vi "LinearQuadraticRegulator_Calculate_NextR.vi"(9 "NextR":T1, 10 "X":T1, 11 "in LinearQuadraticRegulator":T2) -> (0 "Error":bool, 2 "U":T1, 3 "out LinearQuadraticRegulator":T2)   [LabVIEW 2019, in "Trajectory_Library.lvlib"]
doc: "Creates a new LINEAR SYSTEM data cluster with the specified values. \n\n\nInputs: \n - XXX -- XXX.\n\nOutputs:\n - XXX -- XXX."
uses:
  Trajectory_Library.lvlib
  LINEAR_QUADRATIC_REGULATOR.ctl
  <vilib>/Analysis/Matrix/Datatypes/RealMatrix.ctl
  <vilib>/Analysis/Matrix/NI_Matrix.lvlib
panel:
  # "Ref State <States,1>"
  # "Comp and capped \noutput <Inputs,1>"
  # "Controller gain\n<Inputs,States>"
  # "Ref State <States,1>"
  # "Comp and capped \noutput <Inputs,1>"
  # "Controller gain\n<Inputs,States>"
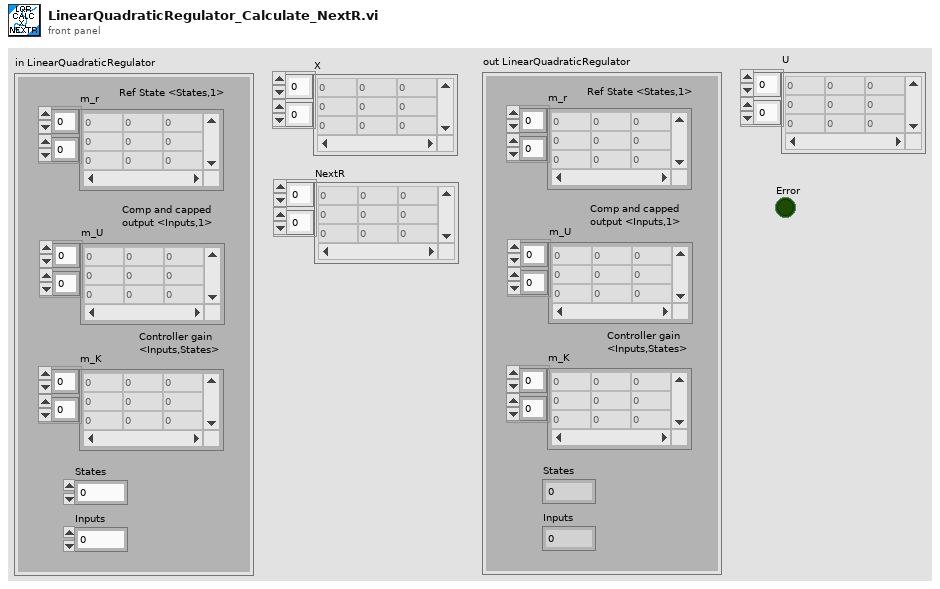
[diagram p1: front panel]
types:
  T1 = typedef "NI_Matrix.lvlib/RealMatrix.ctl" = dbl[][]
  T2 = typedef "Trajectory_Library.lvlib/LINEAR_QUADRATIC_REGULATOR.ctl" = cluster{"m_r":T1, "m_U":T1, "m_K":T1, "States":i32, "Inputs":i32}
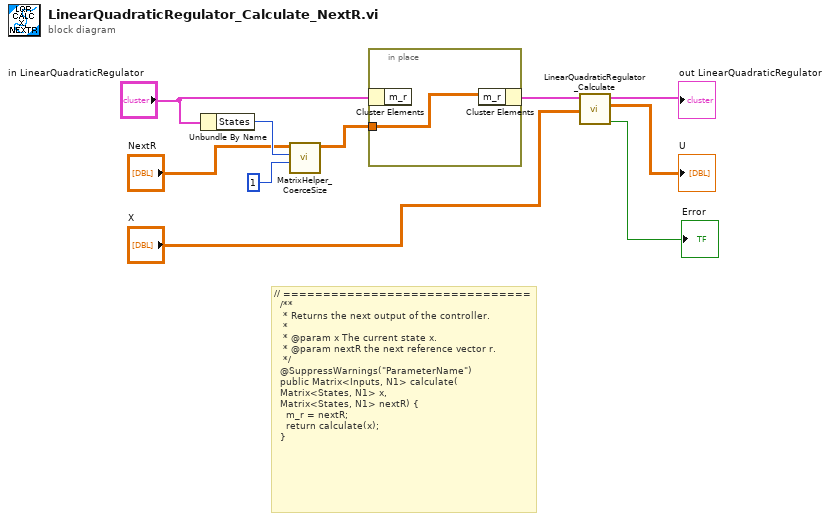
[diagram p0: block diagram]
diagram:
  # "// ===============================\n  /**\n   * Returns the next output of the controller.\n   *\n   * @param x The current state x.\n   * @param nextR the next reference vector r.\n   */\n  @SuppressWarnings(\"ParameterName\")\n  public Matrix<Inputs, N1> calculate(\n\t\tMatrix<States, N1> x, \n\t\tMatrix<States, N1> nextR) {\n    m_r = nextR;\n    return calculate(x);\n  }"
  n1 = Unbundle By Name("in LinearQuadraticRegulator") -> ("States"=w4:i32)
  n2 = call "MatrixHelper_CoerceSize.vi"("Columns"=1 ("y"), "Rows"=w4, "input matrix"="NextR") -> ("output matrix"=w2:T1)  [unwired: 8 in]
  n3 = in-place {
    in-place-border: w2 -> [w11]
    n4 = in-place-cluster #1("in LinearQuadraticRegulator") -> ()  [unwired: 1 out]
    n5 = in-place-cluster #1("m_r"=w11) -> (w9:T2)
  }
  n6 = call "LinearQuadraticRegulator_Calculate.vi"("X"="X", "in LinearQuadraticRegulator"=w9) -> ("Error"=→"Error":bool, "U"=→"U":T1, "out LinearQuadraticRegulator"=→"out LinearQuadraticRegulator":T2)  [unwired: 7 in]
